vi "KE6514.destructor.vi"(0 "i ref in":refnum<vi>, 5 "error in (no error)":errorcluster) -> (19 "error out":errorcluster)   [LabVIEW 2014, in "KE6514.lvlib"]
doc: "This is the destructor of a class.\n\nLicense Agreement for this software:\n\nCopyright (C)\nGesellschaft für Schwerionenforschung, GSI\nPlanckstr. 1\n64291 Darmstadt\nGermany\n\nContact: D.Beck@gsi.de \n\nThis program is free software; you can redistribute it and/or modify it under the terms of the \nGNU General Public License as published by the Free Software Foundation; either version 2 of \nthe license, or (at your option) any later version.\n\nThis program is distributed in the hope that it will be useful, but WITHOUT ANY WARRANTY; \nwithout even the implied warranty of MERCHANTABILITY or FITNESS FOR A PARTICULAR PURPOSE. See the GNU General License for more details (http://www.gnu.org).\n\nGesellschaft für Schwerionenforschung, GSI\nPlanckstr. 1, 64291 Darmstadt, Germany\nFor all questions and ideas contact: M.Richter@gsi.de, H.Brand@gsi.de or D.Beck@gsi.de.\nLast update: 16-JUN-2004"
uses:
  KE6514.lvlib
  CS_Core/CSApplicationBaseClasses/DeviceBase/DeviceBase.lvlib
  instr.lib/KE6514/KE6514Driver.lvlib
  CSlibraries-extern/DimLVEvent/LVDimInterface/LVDimInterface.lvlib
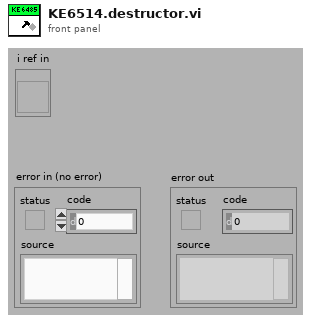
[diagram p1: front panel]
types:
  T1 = typedef "KE6514.lvlib/KE6514.i attribute.ctl" = cluster{"VISA resource name":refnum<visa-resource-name>, "ValueID":i32, "MeasurementRunning?":bool, "actSequencer":string, "actScanner":string, "actPPG":string, "MeasuredID":i32}
  T2 = enum16{"SetAttribute", "GetAttribute", "CreateAttribute", "DestroyAttribute", "DestroyAllAtributes"}
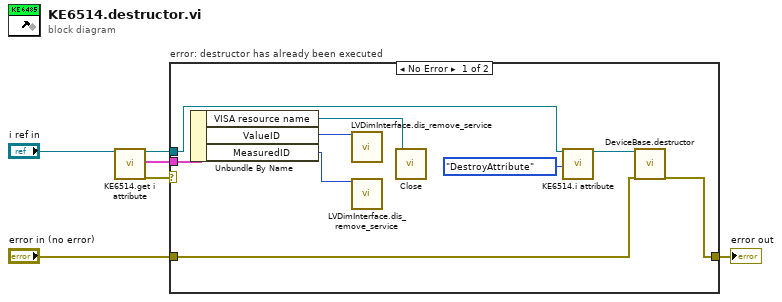
[diagram p0: block diagram]
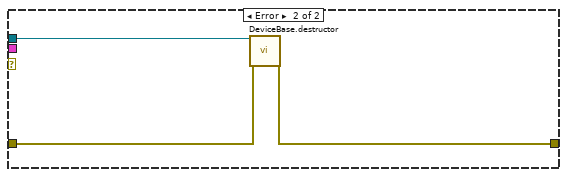
[diagram p2: hidden frame]
diagram:
  n1 = call "KE6514.get i attribute.vi"("i ref in"="i ref in") -> ("i ref out"=w2:refnum<vi>, "i attribute"=w1:T1, "error out"=w3:errorcluster)  [unwired: 16 in]
  n2 = case "error: destructor has already been executed" shown="No Error" w3 {
    tunnel: [w13 w16] -> w6
    tunnel: "error in (no error)" -> [w9 w17]
    tunnel: w2 -> [w10 w18]
    tunnel: w1 -> [w12 _]
    frame No Error {
      n3 = Unbundle By Name(w12) -> ("VISA resource name"=w11:refnum<visa-resource-name>, "ValueID"=w8:i32, "MeasuredID"=w7:i32)
      n4 = call "LVDimInterface.dis_remove_service.vi"("my_serviceID"=w8) -> ()  [unwired: 18 in, 1 out]
      n5 = call "LVDimInterface.dis_remove_service.vi"("my_serviceID"=w7) -> ()  [unwired: 18 in, 1 out]
      n6 = call "Close.vi"("VISA resource name"=w11) -> ()  [unwired: 14 in, 1 out]
      n7 = call "KE6514.i attribute.vi"("VI Refnum"=w10, "Action"=T2."DestroyAttribute") -> ("VI Refnum out"=w14:refnum<vi>)  [unwired: 15 in, 2 out]
      n8 = call "DeviceBase.destructor.vi"("i ref in"=w14, "error in (no error)"=w9) -> ("error out"=w13:errorcluster)  [unwired: 17 in]
    }
    frame Error {
      n9 = call "DeviceBase.destructor.vi"("i ref in"=w18, "error in (no error)"=w17) -> ("error out"=w16:errorcluster)  [unwired: 17 in]
    }
  }
  "error out" <- w6
